vi "IMAQDevice.FindCommand.vi"(1 "Command Array":string[](array[string]), 2 "Sequence Number":i32, 4 "Search String":string) -> (15 "Found Result":string, 17 "Found?":bool)   [LabVIEW 2014, in "IMAQDevice.lvlib"]
uses:
  IMAQDevice.lvlib
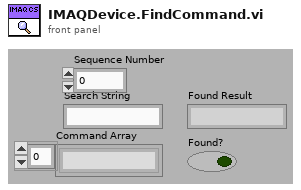
[diagram p1: front panel]
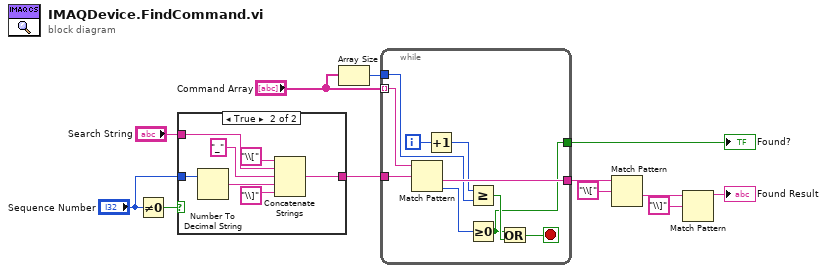
[diagram p0: block diagram]
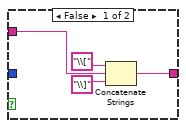
[diagram p2: hidden frame]
diagram:
  n1 = Not Equal To 0?(x="Sequence Number") -> (x != 0?=w3:bool)
  n2 = case shown="True" w3 {
    tunnel: [w13 w23] -> w5
    tunnel: "Search String" -> [w14 w21]
    tunnel: "Sequence Number" -> [_ w20]
    frame False {
      n3 = Concatenate Strings("\\[" ("string"), w14, "\\]" ("string")) -> (w13:string)
    }
    frame True {
      n4 = Number To Decimal String(number=w20) -> (decimal integer string=w17:string)  [unwired: 1 in]
      n5 = Concatenate Strings("\\[" ("string"), w21, "_" ("string"), w17, "\\]" ("string")) -> (w23:string)
    }
  }
  n6 = Array Size(array="Command Array") -> (size(s)=w7:i32)
  n7 = while {
    tunnel: "Command Array" -> [w33] mode=indexing
    tunnel: [w32] -> w11
    tunnel: w7 -> [w26]
    tunnel: w5 -> [w25]
    tunnel: [w24] -> w1
    i -> [w29]
    stop <- w31 stop-if-true
    n8 = Match Pattern(string=w33, regular expression=w25) -> (after substring=w32:string, offset past match=w30:i32)  [unwired: 1 in, 2 out]
    n9 = Increment(x=w29) -> (x+1=w28:i32)
    n10 = Greater Or Equal?(x=w28, y=w26) -> (x >= y?=w27:bool)
    n11 = Greater Or Equal To 0?(x=w30) -> (x >= 0?=w24:bool)
    n12 = Or(x=w24, y=w27) -> (x .or. y?=w31:bool)
  }
  "Found?" <- w1
  n13 = Match Pattern(string=w11, regular expression="\\[") -> (after substring=w9:string)  [unwired: 1 in, 3 out]
  n14 = Match Pattern(string=w9, regular expression="\\]") -> (before substring=→"Found Result":string)  [unwired: 1 in, 3 out]
